vi "Insert Into Subpanel.vi"(7 "Viewable Name":string, 8 "error in (no error)":errorcluster, 9 "Insertion Request Time":timestamp, 10 "VI Refnum":refnum<vi>, 11 "Protected Subpanel":T1) -> (0 "error out":errorcluster, 3 "Protected Subpanel":T1)   [LabVIEW 2015, in "ProtectedSubpanel.lvlib" / "ProtectedSubpanel.lvclass"]
uses:
  ProtectedSubpanel.lvclass
  Protected Subpanel Reference.ctl
  ProtectedSubpanel.lvclass/ProtectedSubpanel.ctl
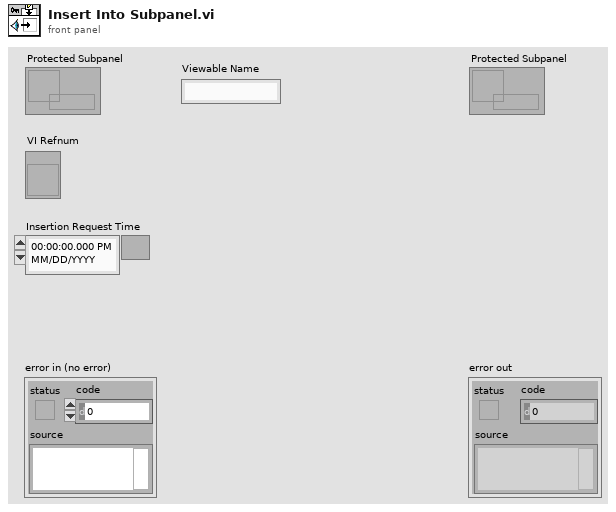
[diagram p1: front panel]
types:
  T1 = typedef "ProtectedSubpanel.lvlib/ProtectedSubpanel.lvclass/Protected Subpanel Reference.ctl" = refnum<data-value>
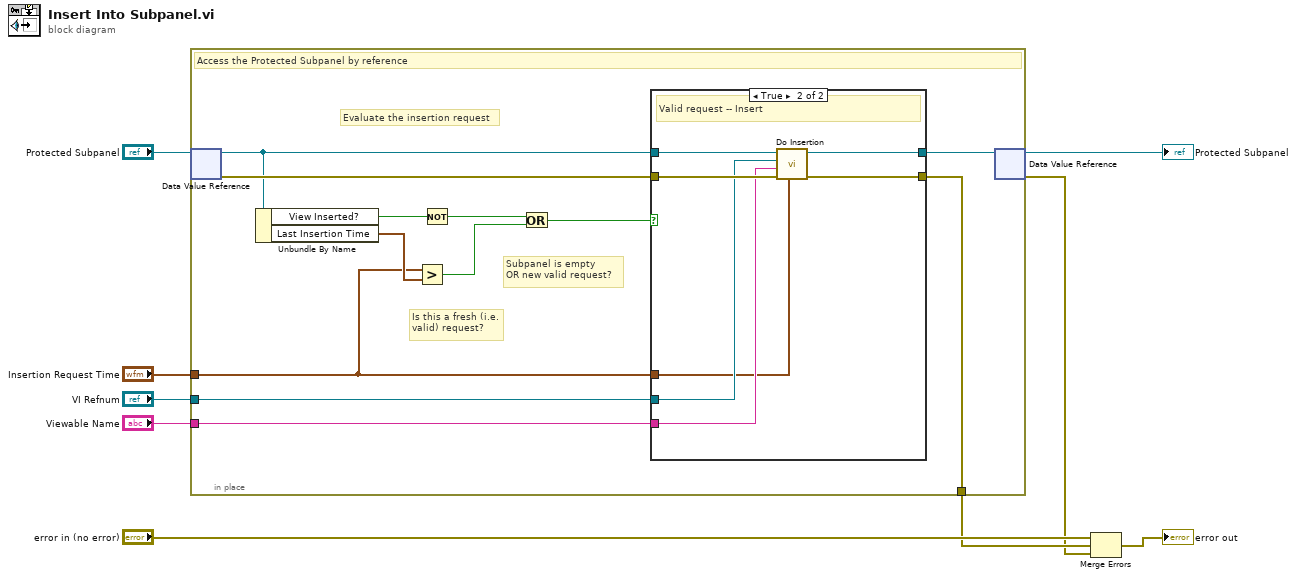
[diagram p0: block diagram]
diagram:
  n1 = in-place {
    in-place-border: "VI Refnum" -> [w20]
    in-place-border: "Insertion Request Time" -> [w10]
    in-place-border: "Viewable Name" -> [w19]
    in-place-border: [w11] -> w2
    # "Evaluate the insertion request"
    # "Subpanel is empty\nOR new valid request?"
    # "Is this a fresh (i.e.\nvalid) request?"
    # "Access the Protected Subpanel by reference"
    n2 = in-place-dvr #1("Protected Subpanel") -> (w12:refnum<class "ProtectedSubpanel.lvclass">, w13:errorcluster)
    n3 = Unbundle By Name(w12) -> ("View Inserted?"=w17:bool, "Last Insertion Time"=w18:timestamp)
    n4 = Greater?(x=w10, y=w18) -> (0:w15:bool)
    n5 = Not(x=w17) -> (.not. x?=w16:bool)
    n6 = Or(x=w16, y=w15) -> (x .or. y?=w14:bool)
    n7 = case shown="True" w14 {
      tunnel: [w23 w30] -> w21
      tunnel: w12 -> [w23 w29]
      tunnel: w13 -> [w22 w28]
      tunnel: [w22 w27] -> w11
      tunnel: w20 -> [_ w26]
      tunnel: w19 -> [_ w25]
      tunnel: w10 -> [_ w24]
      frame False {
        # "Stale request -- No insert"
      }
      frame True {
        # "Valid request -- Insert"
        n8 = call "Do Insertion.vi"("Last Insertion Time"=w24, "error in (no error)"=w28, "View Name"=w25, "VI Refnum"=w26, "ProtectedSubpanel in"=w29) -> ("error out"=w27:errorcluster, "ProtectedSubpanel out"=w30:refnum<class "ProtectedSubpanel.lvclass">)  [unwired: 5 in]
      }
    }
    n9 = in-place-dvr #1(w21) -> (→"Protected Subpanel":T1, w1:errorcluster)
  }
  n10 = Merge Errors("error in (no error)", w2, w1) -> (→"error out":errorcluster)
